vi "Wheel of Doom Get Closest Slot.vi"(9 "Next Full Slot? (F)":bool, 10 "Slot States":T1[](array[typedef]), 11 "Raw Angle":dbl) -> (1 "None Available?":bool, 2 "Angle":dbl, 3 "Slot":i32)   [LabVIEW 2019]
uses:
  Wheel of Doom Slot State.ctl
panel:
  # "0"
  # "1"
  # "2"
  # "3"
  # "4"
  # "5"
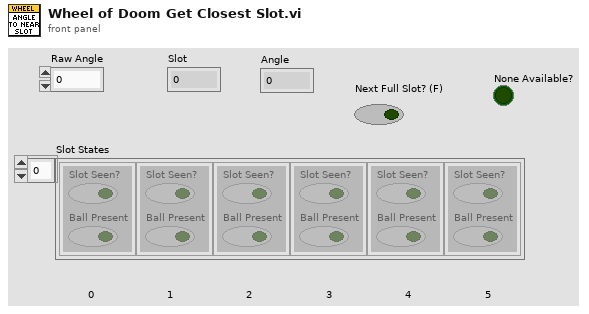
[diagram p1: front panel]
types:
  T1 = typedef "Wheel of Doom Slot State.ctl" = cluster{"Slot Seen?":bool, "Ball Present":bool}
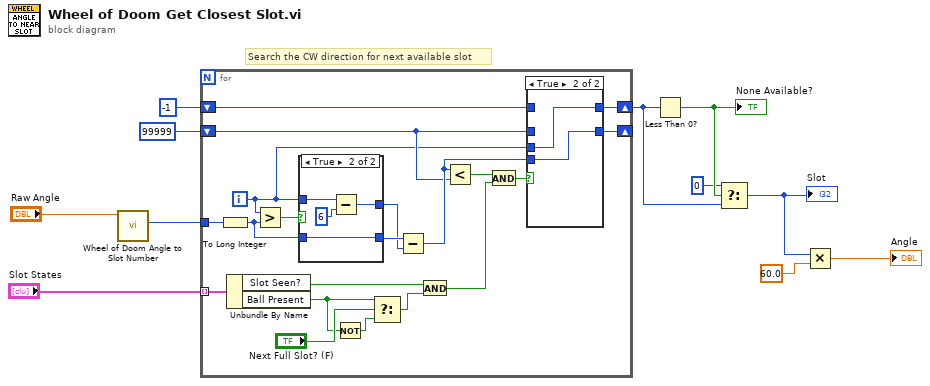
[diagram p0: block diagram]
diagram:
  # "Search the CW direction for next available slot"
  n1 = call "Wheel of Doom Angle to Slot Number.vi"("Sensor Position"="Raw Angle") -> ("Slot Number"=w9:u32)  [unwired: 9 in, 1 out]
  n2 = for {
    tunnel: "Slot States" -> [w31] mode=indexing
    tunnel: w9 -> [w29]
    shift-right: [w20] -> w1
    shift-left: -1 ("y") -> [w18]
    shift-right: [w24] -> _
    shift-left: 99999 ("y") -> [w17]
    i -> [w16]
    n3 = To Long Integer(number=w29) -> (32bit integer=w27:i32)
    n4 = Unbundle By Name(w31) -> ("Slot Seen?"=w30:bool, "Ball Present"=w13:bool)
    n5 = Greater?(x=w16, y=w27) -> (0:w28:bool)
    n6 = case shown="True" w28 {
      tunnel: w16 -> [w37 w41]
      tunnel: w27 -> [w36 w38]
      tunnel: [w37 w39] -> w25
      tunnel: [w36 w38] -> w26
      frame False {
      }
      frame True {
        n7 = Subtract(x=w41, y=6) -> (x-y=w39:i32)
      }
    }
    n8 = Not(x=w13) -> (.not. x?=w14:bool)
    n9 = Select(t=w13, s="Next Full Slot? (F)", f=w14) -> (s? t:f=w12:bool)
    n10 = Subtract(x=w26, y=w25) -> (x-y=w19:i32)
    n11 = And(x=w30, y=w12) -> (x .and. y?=w22:bool)
    n12 = Less?(x=w19, y=w17) -> (x < y?=w23:bool)
    n13 = And(x=w23, y=w22) -> (x .and. y?=w21:bool)
    n14 = case shown="True" w21 {
      tunnel: w16 -> [_ w35]
      tunnel: [w32 w34] -> w24
      tunnel: [w33 w35] -> w20
      tunnel: w19 -> [_ w34]
      tunnel: w18 -> [w33 _]
      tunnel: w17 -> [w32 _]
      frame False {
      }
      frame True {
      }
    }
  }
  n15 = Less Than 0?(x=w1) -> (x < 0?=w6:bool)
  "None Available?" <- w6
  n16 = Select(t=0, s=w6, f=w1) -> (s? t:f=w4:i32)
  "Slot" <- w4
  n17 = Multiply(x=w4, y=60.0) -> (x*y=→"Angle":dbl)
